vi "Omni-Driver-Fast-Open.vi"() -> (0 "Number of Spectrometers":i32, 2 "Wrapper Out":u32)   [LabVIEW 2014]
doc: "André Romero - 2016\nandretec@ifsc.usp.br"
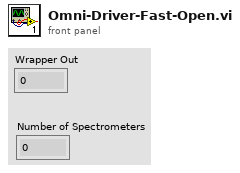
[diagram p1: front panel]
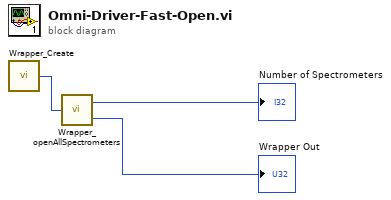
[diagram p0: block diagram]
diagram:
  n1 = call "Wrapper_Create.vi"() -> ("Wrapper"=w3:u32)
  n2 = call "Wrapper_openAllSpectrometers.vi"("Wrapper In"=w3) -> ("Number of Spectrometers"=→"Number of Spectrometers":i32, "Wrapper Out"=→"Wrapper Out":u32)
